vi "demo_Prevent Executing Untrusted VIs.vi"(11 "Stop Demo":refnum<user-event>) -> ()   [LabVIEW 2020]
panel:
  # "LabVIEW 2026 Q1 - Prevent Executing Untrusted VIs\n\nBy default, LabVIEW now prevents unknown external code (i.e. VIs downloaded from the internet) from automatically executing when called or loaded. External code loaded in LabVIEW now loads in a broken, viewable state. You must add external files to the LabVIEW trusted files list using the Manage Trusted Files dialog."
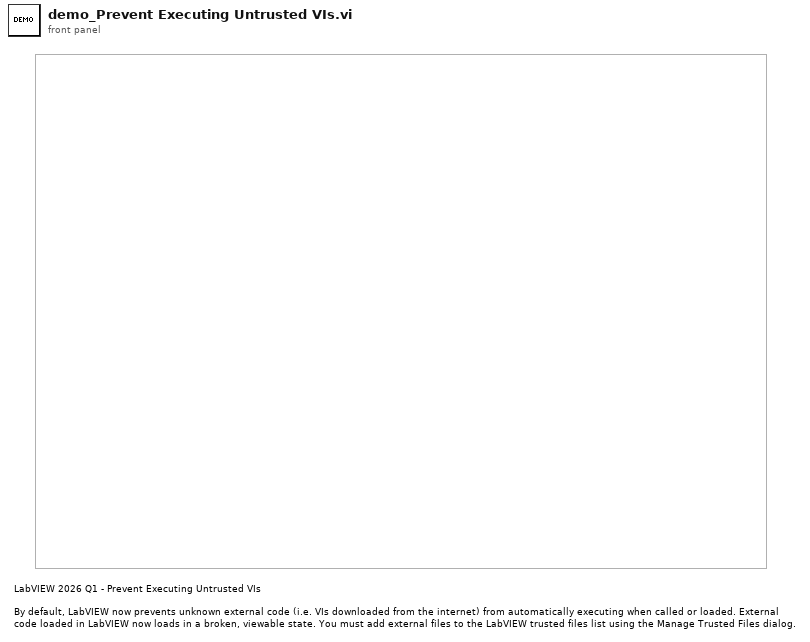
[diagram p1: front panel]
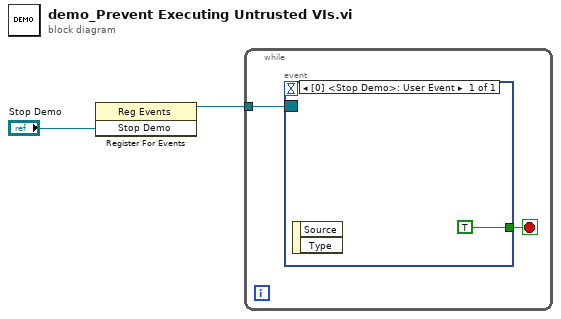
[diagram p0: block diagram]
diagram:
  n1 = register-events("Stop Demo") -> (reference out=w1:refnum<event-registration>)  [unwired: 2 in, 1 out]
  n2 = while {
    tunnel: w1 -> [w4]
    stop <- w3 stop-if-true
    n3 = event shown="[0] <Stop Demo>: User Event" {
      selector: w4 -> [_]
      dyn-events: _ -> [_]
      timeout: _ -> [_]
      tunnel: [TRUE] -> w3
      event User Event {
        n4 = event-data() -> ()  [unwired: 1 in, 2 out]
      }
    }
  }
